vi "Parallel VIs Launcher.vi"   [LabVIEW 2013]
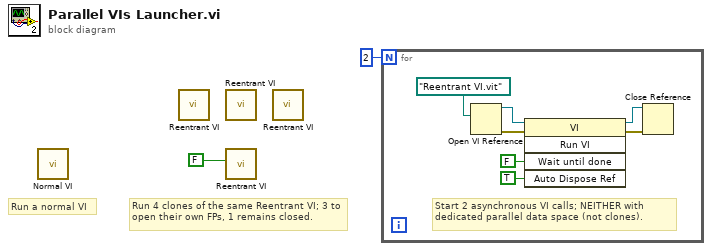
[diagram p0: block diagram]
diagram:
  # "Run a normal VI"
  # "Run 4 clones of the same Reentrant VI; 3 to open their own FPs, 1 remains closed."
  n1 = call "Normal VI.vi"() -> ()  [unwired: 12 in]
  n2 = call "Reentrant VI.vi"() -> ()  [unwired: 12 in]
  n3 = call "Reentrant VI.vi"() -> ()  [unwired: 12 in]
  n4 = call "Reentrant VI.vi"("Open FP? (T)"=FALSE ("Open FP?")) -> ()  [unwired: 11 in]
  n5 = call "Reentrant VI.vi"() -> ()  [unwired: 12 in]
  n6 = for {
    N: 2 -> [_]
    # "Start 2 asynchronous VI calls; NEITHER with dedicated parallel data space (not clones)."
    n7 = Open VI Reference(vi path=path "Reentrant VI.vit") -> (vi reference=w9:refnum<vi>, error out=w8:errorcluster)  [unwired: 5 in]
    n8 = invoke class="VI" method="Run VI"(reference=w9, error in=w8, "Wait until done"=FALSE ("Wait Until Done"), "Auto Dispose Ref"=TRUE ("Auto Dispose Reference")) -> (reference out=w5:refnum<vi>, error out=w4:errorcluster)  [unwired: 1 in, 3 out]
    n9 = Close Reference(reference=w5, error in (no error)=w4) -> ()  [unwired: 1 out]
  }
